vi "Address Space Size.vi"(2 "niUSRP Rx Core v1 FPGA":refnum<class "niUSRP Stream Control (DMA) v1 FPGA.lvclass">) -> (6 "size":u32)   [LabVIEW 2025, in "niUSRP Stream Control (DMA) v1 FPGA.lvclass"]
uses:
  niUSRP Stream Control (DMA) v1 FPGA.lvclass
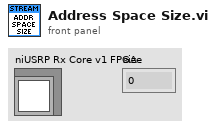
[diagram p1: front panel]
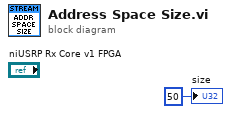
[diagram p0: block diagram]
diagram:
  "size" <- u32 50 ("size")
